vi "GitInit.vi"(8 "error in (no error)":errorcluster, 9 "Directory":path=path "", 11 "Git exec":string="git") -> (0 "error out":errorcluster, 1 "Directory out":path, 2 "Response":string, 3 "Git exec out":string="git")   [LabVIEW 2013]
uses:
  GitCmd.vi
  <vilib>/dlg_ctls.llb/Space Constant.vi
  GitUtils/PathtoDirPath.vi
  <vilib>/Platform/system.llb/System Exec.vi
  <vilib>/Utility/error.llb/Error Cluster From Error Code.vi
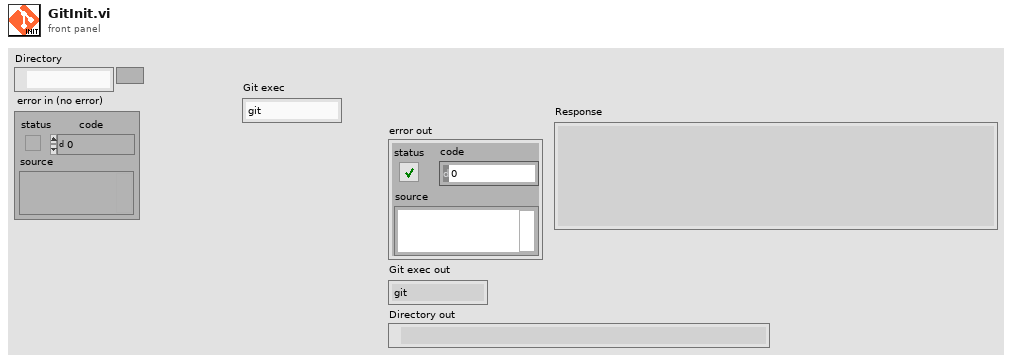
[diagram p1: front panel]
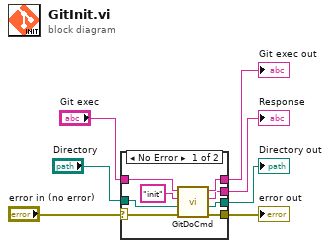
[diagram p0: block diagram]
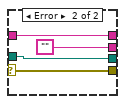
[diagram p2: hidden frame]
diagram:
  n1 = case shown="No Error" "error in (no error)" {
    selector: "error in (no error)" -> [w15 w18]
    tunnel: "Git exec" -> [w12 w16]
    tunnel: "Directory" -> [w14 w17]
    tunnel: [w10 ""] -> w5
    tunnel: [w8 w18] -> w4
    tunnel: [w11 w16] -> w2
    tunnel: [w9 w17] -> w1
    frame No Error {
      n2 = call "GitDoCmd.vi"("error in (no error)"=w15, "Working Path"=w14, "Git command"="init" ("string"), "Git exec"=w12) -> ("error out"=w8:errorcluster, "Working Path out"=w9:path, "Returned stdout"=w10:string, "Git exec out"=w11:string)  [unwired: 3 in]
    }
    frame Error {
    }
  }
  "Response" <- w5
  "error out" <- w4
  "Git exec out" <- w2
  "Directory out" <- w1
